vi "2D kinematics step.vi"(0 "time step (s)":dbl=0.01, 7 "starting 2D state":T1, 11 "2D acceleration (m/s^2)":T3={"x accel (m/s^2)"=9.8, "y accel (m/s^2)"=9.8}) -> (8 "ending 2D state":T1)   [LabVIEW 2016]
doc: "This subvi updates the state of a particle in 2D given the accelaration in 2D and a small time step.\n\nPaul K Dixon\nP350\nCSUSB Physics"
uses:
  typedef/2d state.ctl
  typedef/1d state.ctl
  typedef/2d accel.ctl
panel:
  # "update kinematics in 2D"
  # "update parameters"
  # "Paul K Dixon\nP350"
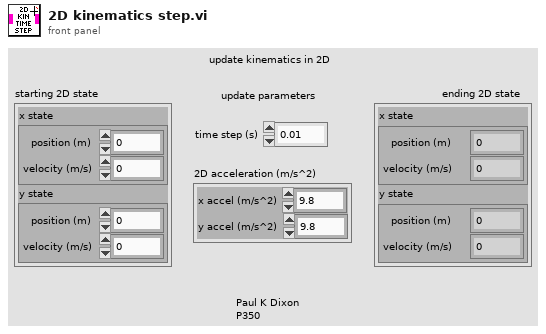
[diagram p1: front panel]
types:
  T1 = typedef "2d state.ctl" = cluster{"x state":T2, "y state":T2}
  T2 = typedef "1d state.ctl" = cluster{"position (m)":dbl, "velocity (m/s)":dbl}
  T3 = typedef "2d accel.ctl" = cluster{"x accel (m/s^2)":dbl, "y accel (m/s^2)":dbl}
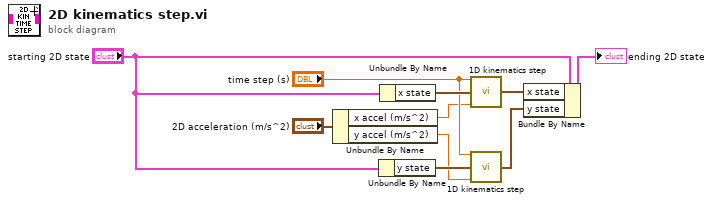
[diagram p0: block diagram]
diagram:
  n1 = Unbundle By Name("2D acceleration (m/s^2)") -> ("x accel (m/s^2)"=w6:dbl, "y accel (m/s^2)"=w1:dbl)
  n2 = Unbundle By Name("starting 2D state") -> ("y state"=w8:T2)
  n3 = Unbundle By Name("starting 2D state") -> ("x state"=w9:T2)
  n4 = call "1D kinematics step.vi"("time step (s)"="time step (s)", "starting state"=w9, "acceleration(m/s^2)"=w6) -> ("ending state"=w5:T2)  [unwired: 12 in]
  n5 = call "1D kinematics step.vi"("time step (s)"="time step (s)", "starting state"=w8, "acceleration(m/s^2)"=w1) -> ("ending state"=w4:T2)  [unwired: 12 in]
  n6 = Bundle By Name(cluster="starting 2D state", "x state"=w5, "y state"=w4) -> (→"ending 2D state":T1)
